vi "NonLinIllumination.vi"(5 "TriggerStart":tag="/Dev3/PFI10", 7 "array curve":dbl[](array[numeric]) format="%0.2f", 8 "error in (no error)":errorcluster, 9 "physical channels":tag="Dev2/ao0", 10 "maximum value":dbl=10.0, 11 "minimum value":dbl) -> (0 "error out":errorcluster, 3 "task out":refnum<k21>)   [LabVIEW 2011]
uses:
  <vilib>/DAQmx/write.llb/DAQmx Write (Analog 1D DBL 1Chan NSamp).vi
  <vilib>/DAQmx/create/channels.llb/DAQmx Create Channel (AO-Voltage-Basic).vi
  <vilib>/DAQmx/configure/timing.llb/DAQmx Timing (Sample Clock).vi
  <vilib>/DAQmx/configure/trigger.llb/DAQmx Start Trigger (Analog Edge).vi
  <vilib>/DAQmx/miscellaneous.llb/DAQmx Fill In Error Info.vi
  Program Files/National Instruments/LabVIEW 2011/resource/objmgr/daqmx.rc
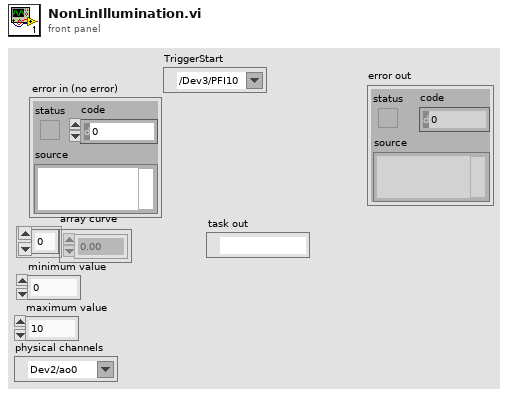
[diagram p1: front panel]
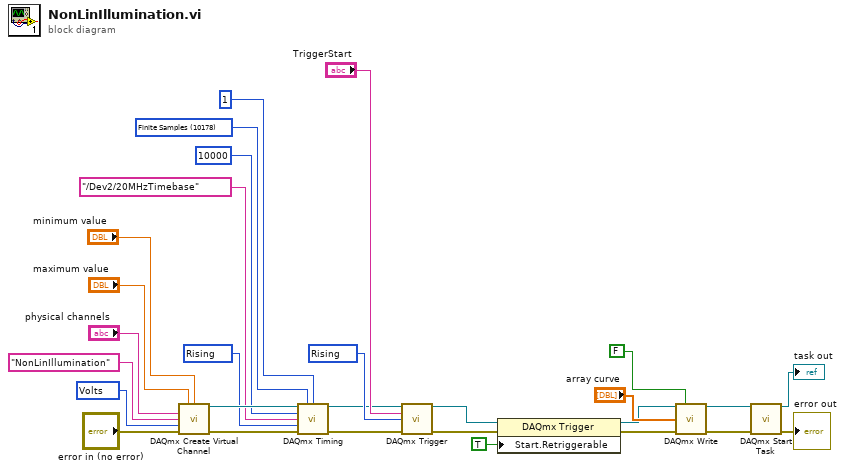
[diagram p0: block diagram]
diagram:
  w13 = 10280 items=["Rising"=10280, "Falling"=10171] ("edge")
  w19 = 10280 items=["Rising"=10280, "Falling"=10171] ("active edge")
  w17 = 10178 items=["Finite Samples"=10178, "Continuous Samples"=10123, "Hardware Timed Single Point"=12522] ("sample mode")
  w16 = 10348 items=["Volts"=10348, "From Custom Scale"=10065] ("units")
  n1 = call-poly <vilib>:"DAQmx Create Virtual Channel.vi"("maximum value"="maximum value", "minimum value"="minimum value", "physical channels"="physical channels", "name to assign"="NonLinIllumination", "units"=w16, "error in"="error in (no error)") -> ("task out"=w21:refnum<k21>, "error out"=w20:errorcluster)  [unwired: 8 in]
  n2 = call-poly <vilib>:"DAQmx Timing.vi"("task/channels in"=w21, "sample mode"=w17, "samples per channel"=1, "rate"=10000, "source"=tag "/Dev2/20MHzTimebase", "active edge"=w19, "error in"=w20) -> ("task out"=w1:refnum<k21>, "error out"=w6:errorcluster)  [unwired: 7 in]
  n3 = call-poly <vilib>:"DAQmx Trigger.vi"("task/channels in"=w1, "source"="TriggerStart", "slope"=w13, "error in"=w6) -> ("task out"=w7:refnum<k21>, "error out"=w8:errorcluster)  [unwired: 10 in]
  n4 = property class="DAQmx Trigger"(reference=w7, error in=w8, "Start.Retriggerable"=TRUE) -> (reference out=w3:refnum<k21>, error out=w4:errorcluster)
  n5 = call-poly <vilib>:"DAQmx Write.vi"("task/channels in"=w3, "auto start"=FALSE, "data"="array curve", "error in"=w4) -> ("task out"=w2:refnum<k21>, "error out"=w5:errorcluster)  [unwired: 9 in, 1 out]
  n6 = call <vilib>:"DAQmx Start Task.vi"("task/channels in"=w2, "error in"=w5) -> ("task out"=→"task out":refnum<k21>, "error out"=→"error out":errorcluster)  [unwired: 12 in]
